vi "ChopperControl.vi"() -> ()   [LabVIEW 2017, in "LIAinteraction.lvlib"]
uses:
  support/LIAinteraction/LIAinteraction.lvlib
  <instrlib>/Stanford Research SR865/Stanford Research SR865.lvlib
panel:
  out "String":string
  in  "Run VI":bool=TRUE
  in  "Chopper Frequency":dbl(knob) scale=0.0..10.0
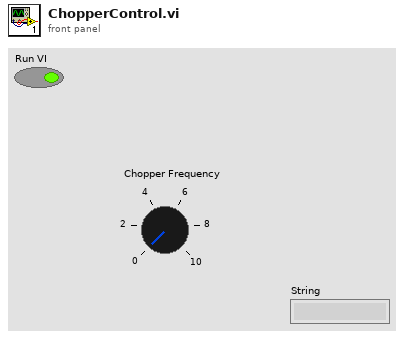
[diagram p1: front panel]
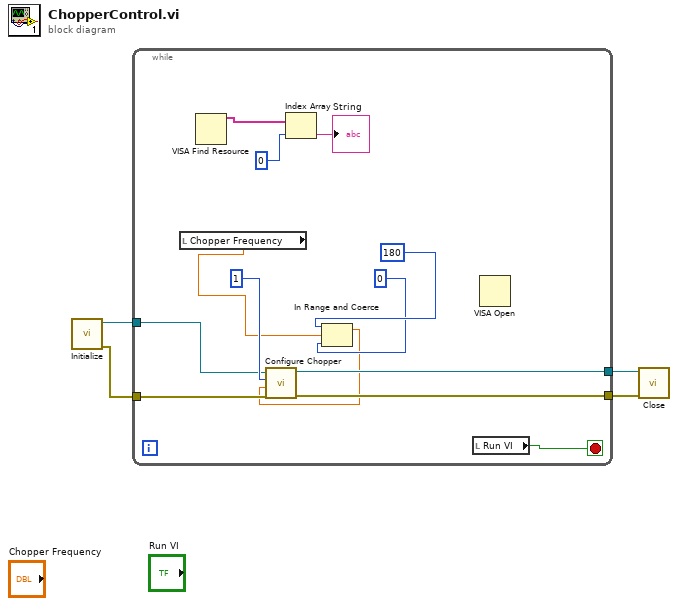
[diagram p0: block diagram]
diagram:
  n1 = call <instrlib>:"Initialize.vi"() -> ("error out"=w2:errorcluster, "VISA resource name out"=w1:refnum<visa-resource-name>)  [unwired: 10 in]
  n2 = while {
    tunnel: [w16] -> w4
    tunnel: [w15] -> w3
    tunnel: w2 -> [w13]
    tunnel: w1 -> [w12]
    stop <- w14 stop-if-true
    n3 = local read "Chopper Frequency"() -> (w9:dbl)
    n4 = VISA Find Resource() -> (3:w7:string[])  [unwired: 3 in, 2 out]
    n5 = Index Array(array=w7, index=0) -> (element=→"String":string)
    n6 = In Range and Coerce(upper limit=180, x=w9, lower limit=0) -> (coerced(x)=w8:dbl)  [unwired: 1 out]
    n7 = call <instrlib>:"Configure Chopper.vi"("error in (no error)"=w13, "Blade Phase (0 Degree)"=w8, "Chopper Blade (0: 6-slot)"=1, "VISA resource name"=w12) -> ("error out"=w16:errorcluster, "VISA resource name out"=w15:refnum<visa-resource-name>)  [unwired: 6 in]
    n8 = local read "Run VI"() -> (w14:bool)
    n9 = VISA Open() -> ()  [unwired: 5 in, 2 out]
  }
  n10 = call <instrlib>:"Close.vi"("error in (no error)"=w4, "VISA resource name"=w3) -> ()  [unwired: 9 in, 1 out]
